vi "Get Module Template Path.vi"(8 "error in (no error)":errorcluster, 11 "Module in":refnum<class "Module.lvclass">) -> (0 "error out":errorcluster, 3 "Module out":refnum<class "Module.lvclass">)   [LabVIEW 2015, in "Module.lvclass"]
uses:
  Module.lvclass
  Module Configuration.ctl
  Module.lvclass/Module.ctl
  Loop/Module Loop/Module Loop.lvclass
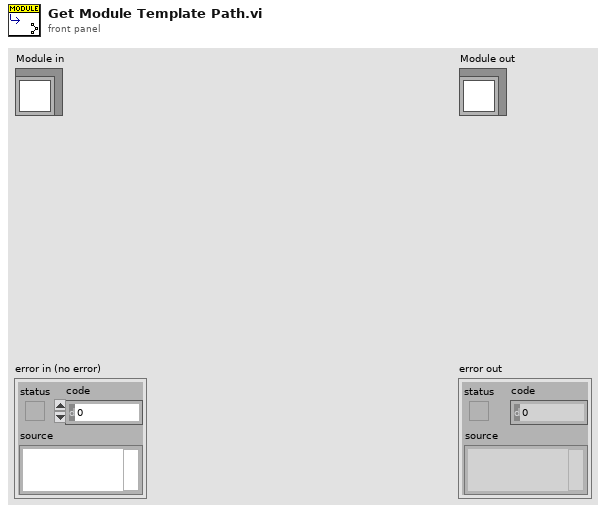
[diagram p1: front panel]
types:
  T1 = typedef "Module Loop.lvclass/Module Configuration.ctl" = cluster{"Type":string, "Direction":string, "Speed":string, "Channels":string, "FXP Type":string}
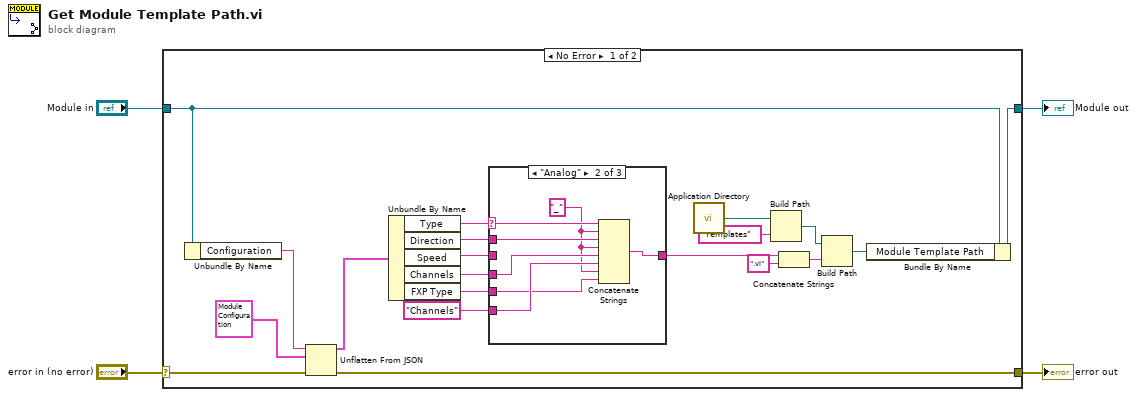
[diagram p0: block diagram]
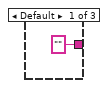
[diagram p2: hidden frame]
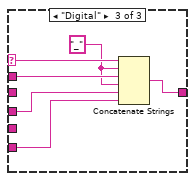
[diagram p3: hidden frame]
diagram:
  n1 = case shown="No Error" "error in (no error)" {
    selector: "error in (no error)" -> [w18 w40]
    tunnel: [w17 w40] -> w3
    tunnel: [w24 w39] -> w1
    tunnel: "Module in" -> [w23 w39]
    frame No Error {
      n2 = Unbundle By Name(w23) -> ("Configuration"=w19:string)
      n3 = Unflatten From JSON(JSON string=w19, type and defaults=T1 {"Type"="Digital", "Direction"="Input", "Speed"="High Speed", "Channels"="8", "FXP Type"=""} ("Cluster"), error in (no error)=w18) -> (value=w15:T1, error out=w17:errorcluster)  [unwired: 4 in]
      n4 = Unbundle By Name(w15) -> ("Type"=w14:string, "Direction"=w13:string, "Speed"=w12:string, "Channels"=w11:string, "FXP Type"=w9:string)
      n5 = case shown="\"Analog\"" w14 {
        selector: w14 -> [_ w32 w38]
        tunnel: w13 -> [_ w31 w37]
        tunnel: w12 -> [_ _ _]
        tunnel: w11 -> [_ w30 w36]
        tunnel: "Channels" ("string") -> [_ w29 w35]
        tunnel: w9 -> [_ w27 _]
        tunnel: ["" w26 w33] -> w8
        frame Default {
        }
        frame "Analog" {
          w28 = "_" ("string")
          n6 = Concatenate Strings(w32, w28, w31, w28, w30, w29, w28, w27) -> (w26:string)
        }
        frame "Digital" {
          w34 = "_" ("string")
          n7 = Concatenate Strings(w38, w34, w37, w34, w36, w35) -> (w33:string)
        }
      }
      n8 = call <vilib>:"Application Directory.vi"() -> ("Application Directory"=w7:path)
      n9 = Build Path(base path=w7, name or relative path="Templates") -> (appended path=w5:path)
      n10 = Concatenate Strings(w8, ".vi" ("string")) -> (w22:string)
      n11 = Build Path(base path=w5, name or relative path=w22) -> (appended path=w20:path)
      n12 = Bundle By Name(cluster=w23, "Module Template Path"=w20) -> (w24:refnum<class "Module.lvclass">)
    }
    frame Error {
    }
  }
  "error out" <- w3
  "Module out" <- w1
